vi "New Panel.vi"() -> ()   [LabVIEW 2012]
uses:
  Type Defs/Alt Control.ctl
  Type Defs/Alt Digit 100 New.ctl
  Type Defs/Alt Display Large.ctl
  Type Defs/All Timers.ctl
  Type Defs/Timer Control.ctl
  Altitude/Altitude.xctl
  Type Defs/Action Time.ctl
  Mode Control/Mode.xctl
  Type Defs/Final Output for Dispaly.ctl
panel:
  in  "Main States":T1(tab)
  out "ALT DISPLAY":T2 format="%#_5f"
  out "Altitude Message":string
  in  "Confirm Now 2":bool
  out "Carbon Dioxide  %":dbl=88890.0
  in  "ALT SET 2":T3 {"Alt Digit 100" min=0 max=9 step=1; "Alt Digit 100" min=0 max=9 step=1; "Alt Digit 100" min=0 max=9 step=1; "Alt Digit 100" min=0 max=9 step=1; "Alt Digit 100" min=0 max=9 step=1}
  in  "Mode 2":cluster{"Run":bool, "Hold":bool, "Off":bool}
  out "ALT DISPLAY 2":T2 format="%#_5f"
  out "Time":string
  in  "Add Note":bool
  out "Final Output Display":T5
  out "CO2 Chart":dbl(graph)
  out "Temp C":dbl=1001.8
  out "Press mB":dbl=1001.8
  out "Date":string
  out "Alt Chart":dbl(graph)
  out "Carbon Dioxide":dbl=88890.0
  in  "Confirm Now":bool
  in  "Notes":string
  in  "ALT SET":T3 {"Alt Digit 100" min=0 max=9 step=1; "Alt Digit 100" min=0 max=9 step=1; "Alt Digit 100" min=0 max=9 step=1; "Alt Digit 100" min=0 max=9 step=1; "Alt Digit 100" min=0 max=9 step=1}
  out "Altitude":dbl=88888.0
  in  "Mode":cluster{"Run":bool, "Hold":bool, "Off":bool}
  in  "Timers":T6 {"Timer 4"."Action Time" format="%<%H:%M>t"; "Timer 3"."Action Time" format="%<%H:%M>t"; "Timer 2"."Action Time" format="%<%H:%M>t"; "Timer"."Action Time" format="%<%H:%M>t"}
  in  "Datalog File":path
  # "Current Effective Altitude in  Meters"
  # "BETA  0.01"
  # "M\nE\nT\nE\nR\nS"
  # "%"
  # "Channel A"
  # "Channel B"
  # "Channel C"
  # "Channel D"
  # "1"
  # "1"
  # "1"
  # "1"
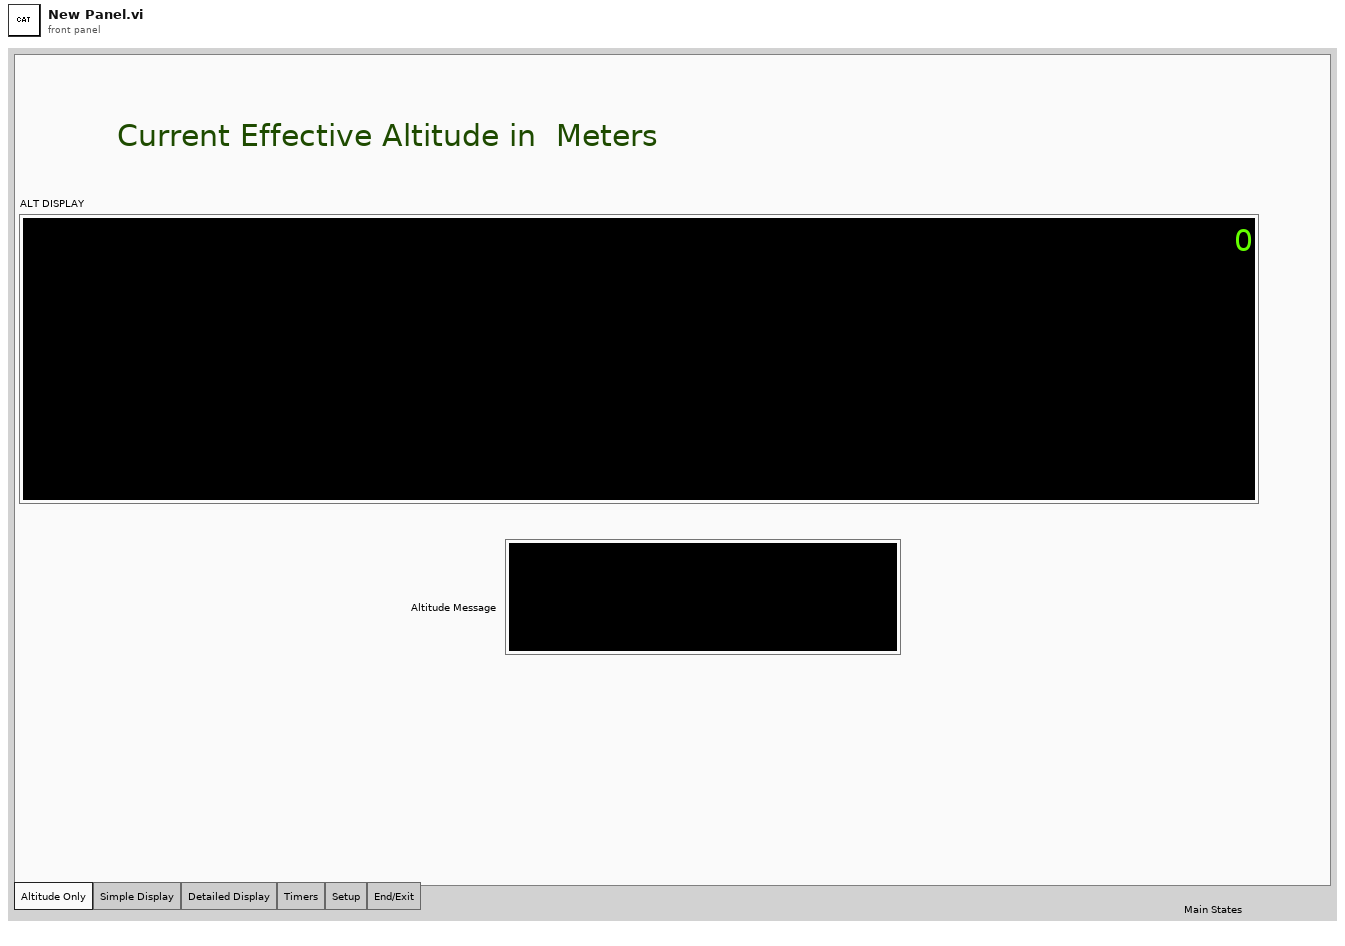
[diagram p1: front panel]
types:
  T1 = enum32{"Altitude Only", "Simple Display", "Detailed Display", "Timers", "Setup", "End/Exit"}
  T2 = typedef "Alt Display Large.ctl" = sgl
  T3 = typedef "Alt Control.ctl" = cluster{"Alt Digit 100":T4, "Alt Digit 100":T4, "Alt Digit 100":T4, "Alt Digit 100":T4, "Alt Digit 100":T4}
  T4 = typedef "Alt Digit 100 New.ctl" = i8
  T5 = typedef "Final Output for Dispaly.ctl" = cluster{"A-1,  1":bool, "A-3,  2":bool, "A-4, 3":bool, "A-5, 4":bool, "ABCD-7, 5":bool, "A-8, 6":bool, "B-1,  7":bool, "B-3, 8":bool, "B-4,  9":bool, "B-5, 10":bool, "B-8, 11":bool, "C-1, 12":bool, "C-3, 13":bool, "C-4, 14":bool, "C-5,  15":bool, "C-8, 16":bool, "A-1, 17":bool, "D-3, 18":bool, "D-4,  19":bool, "D-5,  20":bool, "D-8,  21":bool}
  T6 = typedef "All Timers.ctl" = cluster{"Timer":T7, "Timer 2":T7, "Timer 3":T7, "Timer 4":T7}
  T7 = typedef "Timer Control.ctl" = cluster{"Sun":bool, "Timer":bool, "Altitude":sgl, "Action Time":T8, "Mon":bool, "Tues":bool, "Wed":bool, "Thur":bool, "Fri":bool, "Sat":bool, "Mode":enum8{"Off", "Stby", "Hold", "Run"}}
  T8 = typedef "Action Time.ctl" = dbl
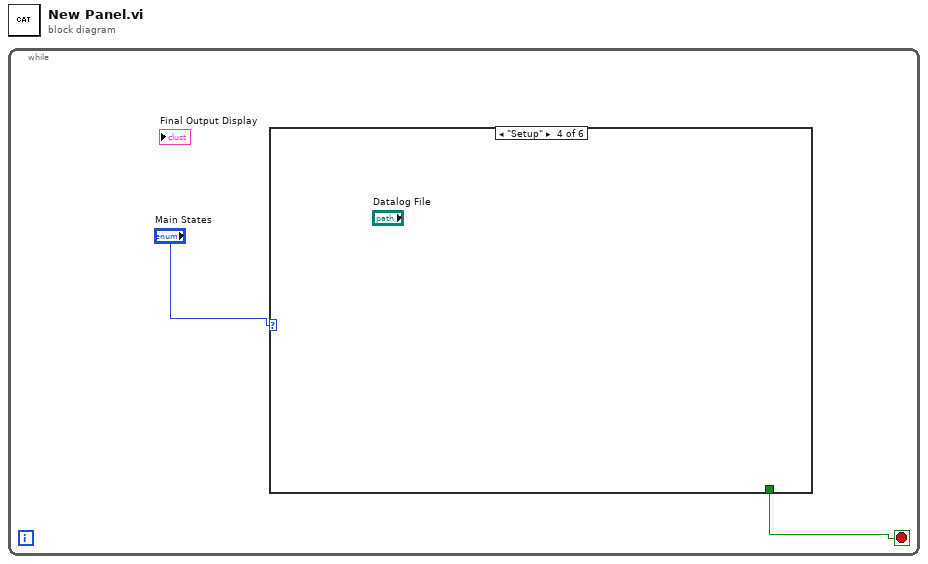
[diagram p0: block diagram]
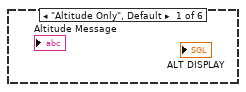
[diagram p2: hidden frame]
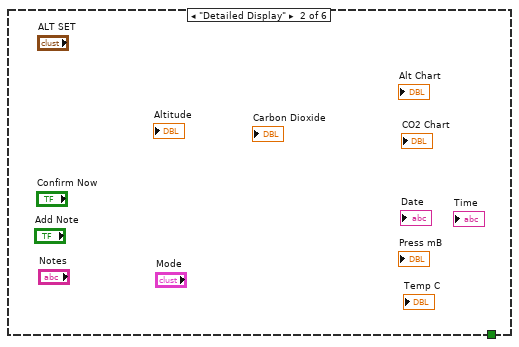
[diagram p3: hidden frame]
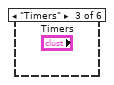
[diagram p4: hidden frame]
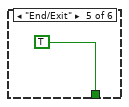
[diagram p5: hidden frame]
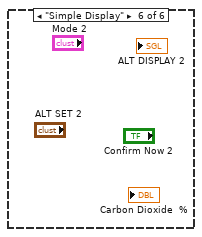
[diagram p6: hidden frame]
diagram:
  n1 = while {
    stop <- w1 stop-if-true
    n2 = case shown="\"Setup\"" "Main States" {
      tunnel: [_ _ _ _ TRUE ("stop") _] -> w1
      frame "Altitude Only", Default {
      }
      frame "Detailed Display" {
      }
      frame "Timers" {
      }
      frame "Setup" {
      }
      frame "End/Exit" {
      }
      frame "Simple Display" {
      }
    }
  }
